vi "Record Path.vi"(9 "Record Path":bool) -> ()   [LabVIEW 2020]
uses:
  Framework/Robot Global Data.vi
  <vilib>/Analysis/Matrix/Numeric/Conversions/Matrix To Array - RM.vi
  <vilib>/Utility/file.llb/Write Delimited Spreadsheet (DBL).vi
  <vilib>/Analysis/Matrix/NI_Matrix.lvlib
panel:
  out "error out":errorcluster
  out "path":path
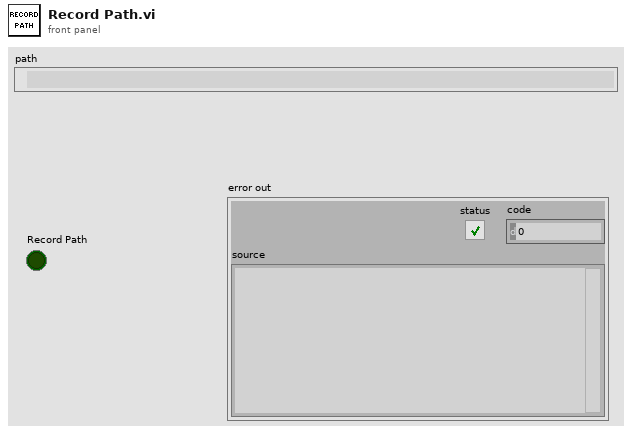
[diagram p1: front panel]
types:
  T1 = typedef "NI_Matrix.lvlib/RealMatrix.ctl" = dbl[][]
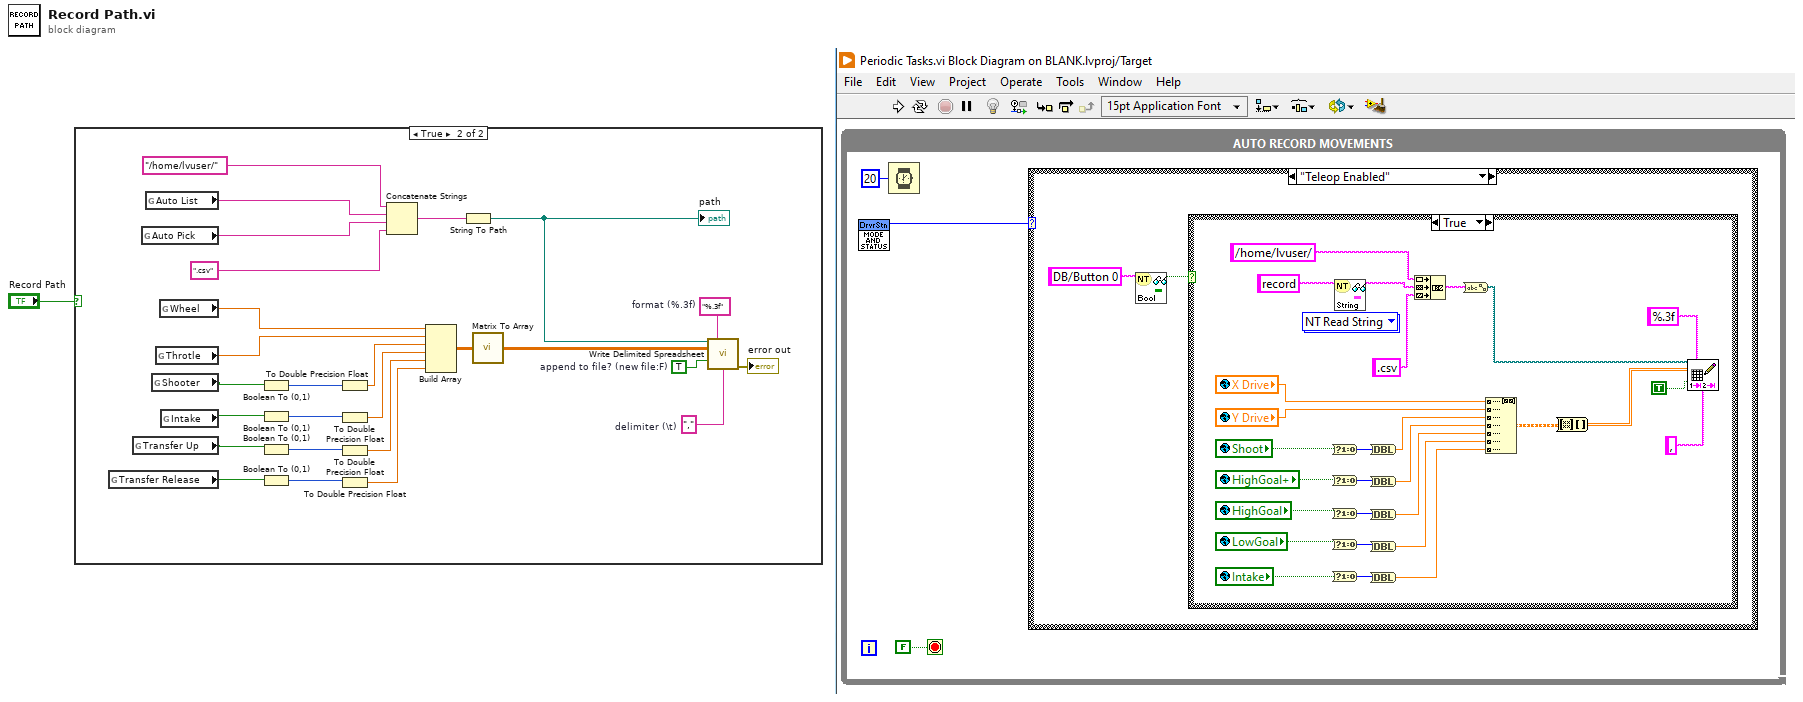
[diagram p0: block diagram]
diagram:
  n1 = case shown="True" "Record Path" {
    frame False {
    }
    frame True {
      w16 = TRUE  # append to file? (new file:F)
      w17 = "%.3f"  # format (%.3f)
      w12 = ","  # delimiter (\t)
      n2 = global read "Robot Global Data.vi" "Transfer Release"() -> (w6:bool)
      n3 = global read "Robot Global Data.vi" "Transfer Up"() -> (w7:bool)
      n4 = global read "Robot Global Data.vi" "Auto Pick"() -> (w4:string)
      n5 = global read "Robot Global Data.vi" "Auto List"() -> (w5:string)
      n6 = global read "Robot Global Data.vi" "Shooter"() -> (w9:bool)
      n7 = global read "Robot Global Data.vi" "Throtle"() -> (w10:dbl)
      n8 = global read "Robot Global Data.vi" "Wheel"() -> (w11:dbl)
      n9 = global read "Robot Global Data.vi" "Intake"() -> (w8:bool)
      n10 = Boolean To (0,1)(Boolean=w9) -> (0, 1=w25:i16)
      n11 = Boolean To (0,1)(Boolean=w8) -> (0, 1=w24:i16)
      n12 = Boolean To (0,1)(Boolean=w7) -> (0, 1=w23:i16)
      n13 = Boolean To (0,1)(Boolean=w6) -> (0, 1=w22:i16)
      n14 = To Double Precision Float(number=w25) -> (double precision float=w21:dbl)
      n15 = To Double Precision Float(number=w24) -> (double precision float=w20:dbl)
      n16 = To Double Precision Float(number=w23) -> (double precision float=w19:dbl)
      n17 = To Double Precision Float(number=w22) -> (double precision float=w18:dbl)
      n18 = Concatenate Strings("/home/lvuser/", w5, w4, ".csv") -> (w13:string)
      n19 = Build Array(w11, w10, w21, w20, w19, w18) -> (w27:T1)
      n20 = String To Path(string=w13) -> (path=w3:path)
      "path" <- w3
      n21 = call-poly <vilib>:"Matrix To Array.vi"("Real Matrix"=w27) -> ("Real 2D Array"=w26:dbl[][])
      n22 = call-poly <vilib>:"Write Delimited Spreadsheet.vi"("file path (dialog if empty)"=w3, "format (%.3f)"=w17, "2D data"=w26, "append to file? (new file:F)"=w16, "delimiter (\\t)"=w12) -> ("error out"=→"error out":errorcluster)  [unwired: 9 in, 1 out]
    }
  }
